vi "Complex Matrix Condition Number.vi"(2 "norm type":T1 items=["2-norm", "1-norm", "F-norm", "Inf-norm"], 3 "Input Matrix":T2) -> (0 "error":i32, 1 "condition number":dbl format="%.4f")   [LabVIEW 2017, in "NI_AALPro.lvlib"]
doc: "Computes the <B>condition number</B> of <B>Input Matrix</B>. Wire data to the <B>Input Matrix</B> input to determine the polymorphic instance to use or manually select the instance."
uses:
  <vilib>/Analysis/NI_AALPro.lvlib
  <vilib>/Analysis/Matrix/Datatypes/ComplexMatrix.ctl
  <vilib>/Analysis/_algsub.llb/Matrix Norm Type.ctl
  <resource>/lvanlys.dll
  <vilib>/Analysis/Matrix/NI_Matrix.lvlib
panel:
  # "Complex\nMatrix Condition Number"
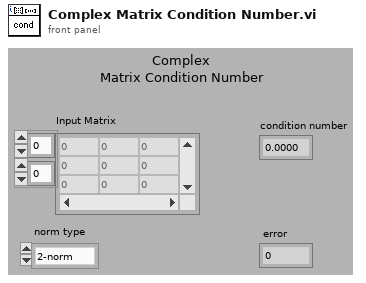
[diagram p1: front panel]
types:
  T1 = typedef "NI_AALPro.lvlib/Matrix Norm Type.ctl" = i32
  T2 = typedef "NI_Matrix.lvlib/ComplexMatrix.ctl" = cdb[][]
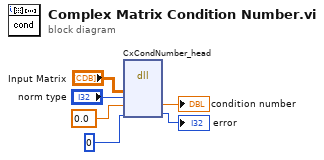
[diagram p0: block diagram]
diagram:
  n1 = dll-call lib="e:/builds/penguin/labview/branches/2017/dev/dist/resource/lvanlys.*" fn="CxCondNumber_head"("Input Matrix"="Input Matrix", "norm type"="norm type", "output param"=0.0, "output param"=0) -> ("output param"=→"condition number":dbl, "output param"=→"error":i32)  [unwired: 6 in, 2 out]
